vi "Spectra_stand_alone.vi"() -> ()   [LabVIEW 2011]
uses:
  <vilib>/Utility/file.llb/Read From Spreadsheet File (DBL).vi
panel:
  out "Waveform Graph 2":dbl[](graph)
  out "Waveform Graph":cluster{"x":dbl, "x":dbl, "all rows":dbl[]}(graph)
  in  "Step size":dbl=0.48
  in  "file path (dialog if empty)":path
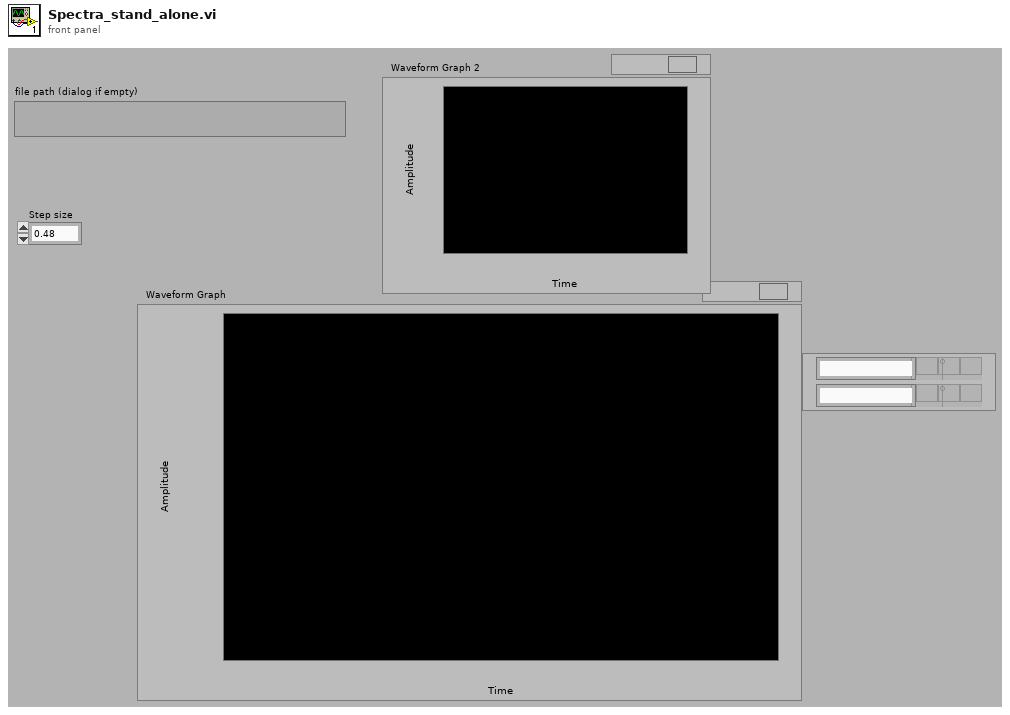
[diagram p1: front panel]
types:
  T1 = cluster{"x":dbl, dbl, "Spectrum output array":dbl[]}
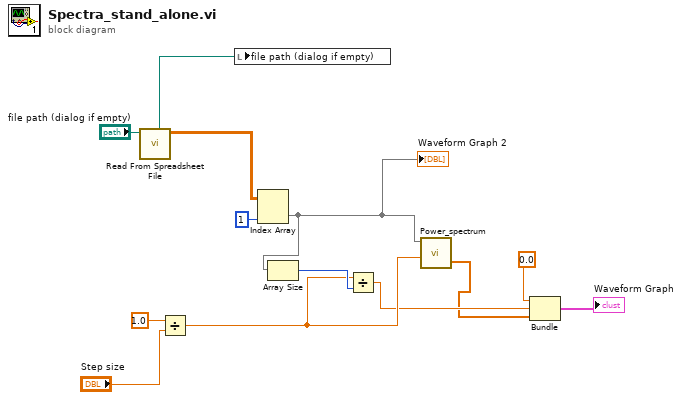
[diagram p0: block diagram]
diagram:
  n1 = call-poly <vilib>:"Read From Spreadsheet File.vi"("file path (dialog if empty)"="file path (dialog if empty)") -> ("all rows"=w11:dbl[][], "new file path (Not A Path if cancelled)"=w12:path)  [unwired: 3 in, 6 out]
  n2 = Divide(x=1.0, y="Step size") -> (x/y=w4:dbl)
  n3 = local write "file path (dialog if empty)"(w12) -> ()
  n4 = Index Array(array=w11, index (col)=1 ("disabled index (col)")) -> (element=w2:dbl[])  [unwired: 1 in]
  "Waveform Graph 2" <- w2
  n5 = Array Size(array=w2) -> (size(s)=w5:i32)
  n6 = Divide(x=w4, y=w5) -> (x/y=w3:dbl)
  n7 = call "Power_spectrum.vi"("U"=w2, "Sampling frequency"=w4) -> ("Spectrum output array"=w1:dbl[])  [unwired: 2 in, 2 out]
  n8 = Bundle("x"=0.0, w3, "Spectrum output array"=w1) -> (→"Waveform Graph":T1)  [unwired: 1 out]
